vi "ATS_AutoCalibrate.vi"(11 "DeviceIn":i32) -> (0 "Return Code":u32, 3 "DeviceOut":i32, 5 "#Device":i32)   [LabVIEW 2015]
doc: "_____AlazarTech, Scope_____\n\nPerform a board specific calibration.\n\nInput:\n\"DeviceIn\" = board to do the calibration\n\nOutput:\n\"#Device\"= number of board in system\n\"DeviceOut\" = duplicate of deviceIn\n\"Return Code\" = status code"
uses:
  ATS_ctl/ATS_Global_Ctrl.ctl
  ATSApi.dll
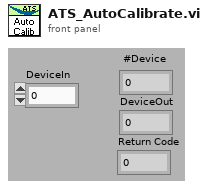
[diagram p1: front panel]
types:
  T1 = typedef "ATS_Global_Ctrl.ctl" = enum16{"Init_Device", "Clear_ALL", "Set", "Get"}
  T2 = typedef "Device_Info.ctl" = cluster{"Handle":u32, "Board":string, "CPLD":string, "MemorySize":u32, "SampleSize":u8, "ID":i32, "High_Memory":bool, "Chan/Board":u8}
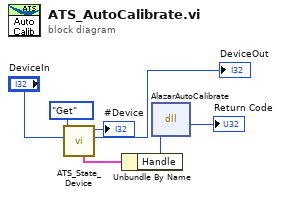
[diagram p0: block diagram]
diagram:
  n1 = call "ATS_State_Device.vi"("DeviceIn"="DeviceIn", "ATS_GBL_Ctrl"=ATS_Global_Ctrl."Get") -> ("DeviceOut"=→"DeviceOut":i32, "#Device"=→"#Device":i32, "DevInfo_Out"=w2:T2)  [unwired: 4 in, 3 out]
  n2 = Unbundle By Name(w2) -> ("Handle"=w5:u32)
  n3 = dll-call lib="C:/IntensityOCT/trunk/ATSApi.*" fn="AlazarAutoCalibrate"("h"=w5) -> (→"Return Code":u32)  [unwired: 4 in, 2 out]
